vi "STAV Close.vi"(8 "error in (no error)":errorcluster, 11 "STAV ref in":refnum<visa-resource-name>) -> (0 "error out":errorcluster)   [LabVIEW 2021, in "STAV lib.lvlib"]
uses:
  STAV lib.lvlib
  STAV CommandList.ctl
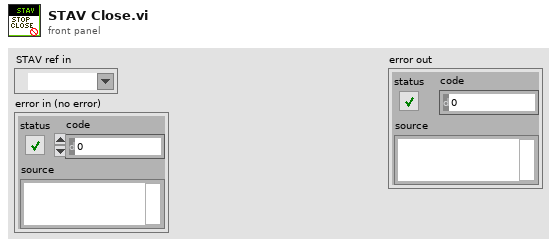
[diagram p1: front panel]
types:
  T1 = typedef "STAV lib.lvlib/STAV CommandList.ctl" = enum16{"StartSending (0)", "StopSending(0)", "FindHomePos(0)", "SetSendingConfig(2)", "GetSendingConfig(0)", "SetPosition(2)", "SetSpeed(2)", "GetSpeed(0)", "GetPosition(0)", "GetForce(0)", "GetPeak(0)", "GetPeakDistance(0)", "GetTravelDistance(0)", "ResetTravelDistance(0)", "GetCycleNo(0)", "GetStepNo(0)", "GetDuration(0)", "GetProfilePosition(0)", "GetHoldTime(0)", "Stop(0)", "StartAndSend(0)", "Start(0)", "Reset(0)", "GetActiveProfile(0)", "SetActiveProfile(2)", "GetProfileCnt(1)", "GetMaxStepCnt(1)", "GetStepCnt(2)", "GetProfileIndex(2)", "SetProfile(3)", "SetStep(3+params)", "GetProfile(2)", "GetStep(3)", "SetProfile(2+params)", ""}
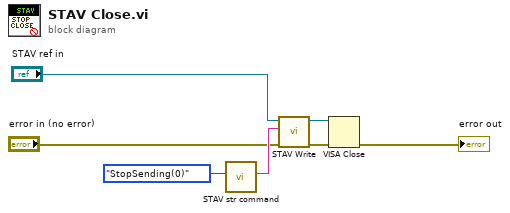
[diagram p0: block diagram]
diagram:
  n1 = call "STAV str command.vi"("Command"=STAV_CommandList."StopSending(0)") -> ("str command"=w3:string)  [unwired: 9 in, 1 out]
  n2 = call "STAV Write.vi"("error in (no error)"="error in (no error)", "Command"=w3, "STAV ref in"="STAV ref in") -> ("error out"=w2:errorcluster, "STAV ref out"=w5:refnum<visa-resource-name>)  [unwired: 7 in]
  n3 = VISA Close(VISA resource name=w5, error in (no error)=w2) -> (error out=→"error out":errorcluster)
